vi "ArgoBot_Read.vi"(10 "Open_Cluster":T8) -> (0 "Analog 3":dbl, 1 "Analog 2":dbl, 2 "Analog 1":dbl, 3 "Read_Value":T9 {"Voltage" scale=0.0..6.5; "Analog 1" format="%#_2g"; "Analog 2" format="%#_2g"; "Analog 3" format="%#_2g"; "Loop Rate (Hz)" scale=0.0..50.0}, 4 "GPIO 1 Read":bool, 5 "GPIO 2 Read":bool, 6 "Read_Cluster":T7, 7 "GPIO 3 Read":bool, 8 "Read_Joystick":T10)   [LabVIEW 2016, in "ArgoBotLib.lvlib"]
uses:
  ArgoBotLib.lvlib
  <vilib>/MakerHub/LINX/Private/Type Defs/LINX Ref.ctl
  <vilib>/MakerHub/LINX/Private/Type Defs/Platform.ctl
  <vilib>/MakerHub/LINX/Private/Type Defs/Interface.ctl
  <vilib>/MakerHub/LINX/Private/Device/Type Defs/LINX Device Config.ctl
  <vilib>/MakerHub/LINX/Private/Device/Type Defs/TCP Config.ctl
  <vilib>/MakerHub/LINX/Private/Device/Type Defs/Channels.ctl
  <vilib>/MakerHub/LINX/LMH-LINX.lvlib
  <vilib>/MakerHub/LINX/Private/Device/Device.lvlib
panel:
  # "ArgoBot  Read"
  # "This vi reads the GPIO and Analog channels"
  # "Outputs"
  # "Inputs"
  # "Battery Voltage"
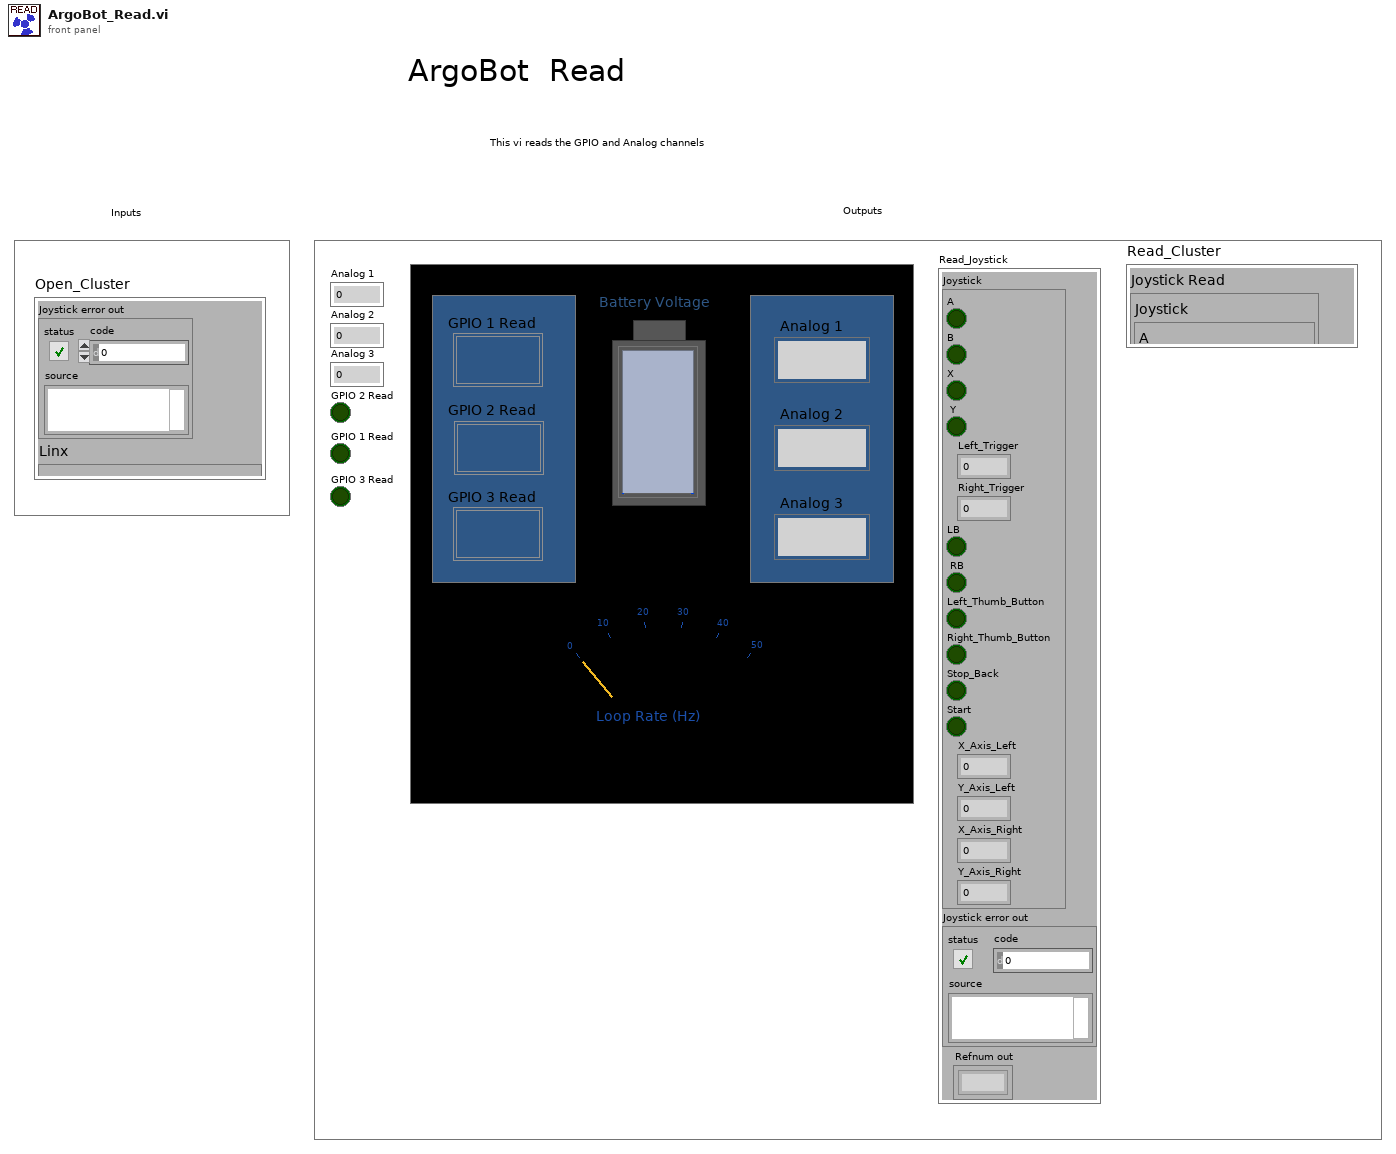
[diagram p1: front panel]
types:
  T1 = typedef "LMH-LINX.lvlib/LINX Ref.ctl" = cluster{"IO":T2, "Interface":T3, "LINX Device Config":T4}
  T2 = typedef "LMH-LINX.lvlib/Platform.ctl" = enum16{"Remote", "Local"}
  T3 = typedef "LMH-LINX.lvlib/Interface.ctl" = enum16{"Serial", "TCP"}
  T4 = typedef "LMH-LINX.lvlib/Device.lvlib/LINX Device Config.ctl" = cluster{"Interface":T3, "COM Port":refnum<visa-resource-name>, "TCP Configuration":T5, "Device Family":u8, "Device ID":u8, "Device Name":string, "TCP Ref":refnum<k5>, "Channels":T6}
  T5 = typedef "LMH-LINX.lvlib/Device.lvlib/TCP Config.ctl" = cluster{"IP Address":string, "Port":u16}
  T6 = typedef "LMH-LINX.lvlib/Channels.ctl" = cluster{"DI":u8[], "DO":u8[], "AI":u8[], "AO":u8[], "PWM":u8[], "QE":u8[], "UART":u8[], "I2C 2":u8[], "SPI":u8[], "CAN":u8[], "Servo":u8[], "AI Ref (V)":dbl, "AI Resolution (Bits)":u8, "AO Ref (V)":dbl, "AO Resolution (Bits)":u8}
  T7 = cluster{"Joystick Read":cluster{"Joystick":cluster{"A":bool, "B":bool, "X":bool, " Y":bool, "Left_Trigger":dbl, "Right_Trigger ":dbl, "LB":bool, " RB":bool, "Left_Thumb_Button":bool, "Right_Thumb_Button":bool, "Stop_Back":bool, "Start":bool, "X_Axis_Left":dbl, "Y_Axis_Left":dbl, "X_Axis_Right":dbl, "Y_Axis_Right":dbl}, "Joystick error out":errorcluster, "Refnum out":refnum<k1>}, "Read Config":cluster{"Read_Config":i32[], "Error Out":errorcluster, "LINX Resource 2":T1}, "Read_Value":cluster{"Analog 1":dbl, "Analog 2":dbl, "Analog 3":dbl, "Voltage":dbl, "GPIO 1 Read":bool, "GPIO 2 Read":bool, "GPIO 3 Read":bool, "Loop Rate (Hz)":u32}, "Joystick error out":errorcluster, "Linx":cluster{"LINX Ref":T1, "Error Out":errorcluster}, "Setup":cluster{"Analog 1 Config":u16, "Analog 2 Config":u16, "Analog 3 Config":u16, "GPIO 1 Config":u16, "GPIO 2 Config":u16, "GPIO 3 Config":u16, "Drive Config":u16, "Motor Mode":u16, "Battery_Config":u16, "LED Config":u16}}
  T8 = cluster{"Joystick error out":errorcluster, "Linx":cluster{"LINX Ref":T1, "Error Out":errorcluster}, "Setup":cluster{"Analog 1 Config":u16, "Analog 2 Config":u16, "Analog 3 Config":u16, "GPIO 1 Config":u16, "GPIO 2 Config":u16, "GPIO 3 Config":u16, "Drive Config":u16, "Motor Mode":u16, "Battery_Config":u16, "LED Config":u16}}
  T9 = cluster{"Analog 1":dbl, "Analog 2":dbl, "Analog 3":dbl, "Voltage":dbl, "GPIO 1 Read":bool, "GPIO 2 Read":bool, "GPIO 3 Read":bool, "Loop Rate (Hz)":u32}
  T10 = cluster{"Joystick":cluster{"A":bool, "B":bool, "X":bool, " Y":bool, "Left_Trigger":dbl, "Right_Trigger ":dbl, "LB":bool, " RB":bool, "Left_Thumb_Button":bool, "Right_Thumb_Button":bool, "Stop_Back":bool, "Start":bool, "X_Axis_Left":dbl, "Y_Axis_Left":dbl, "X_Axis_Right":dbl, "Y_Axis_Right":dbl}, "Joystick error out":errorcluster, "Refnum out":refnum<k1>}
  T11 = cluster{"Read_Config":i32[], "Error Out":errorcluster, "LINX Resource 2":T1}
  T12 = cluster{"A":bool, "B":bool, "X":bool, " Y":bool, "Left_Trigger":dbl, "Right_Trigger ":dbl, "LB":bool, " RB":bool, "Left_Thumb_Button":bool, "Right_Thumb_Button":bool, "Stop_Back":bool, "Start":bool, "X_Axis_Left":dbl, "Y_Axis_Left":dbl, "X_Axis_Right":dbl, "Y_Axis_Right":dbl}
  T13 = cluster{"Analog 1 Config":u16, "Analog 2 Config":u16, "Analog 3 Config":u16, "GPIO 1 Config":u16, "GPIO 2 Config":u16, "GPIO 3 Config":u16, "Drive Config":u16, "Motor Mode":u16, "Battery_Config":u16, "LED Config":u16}
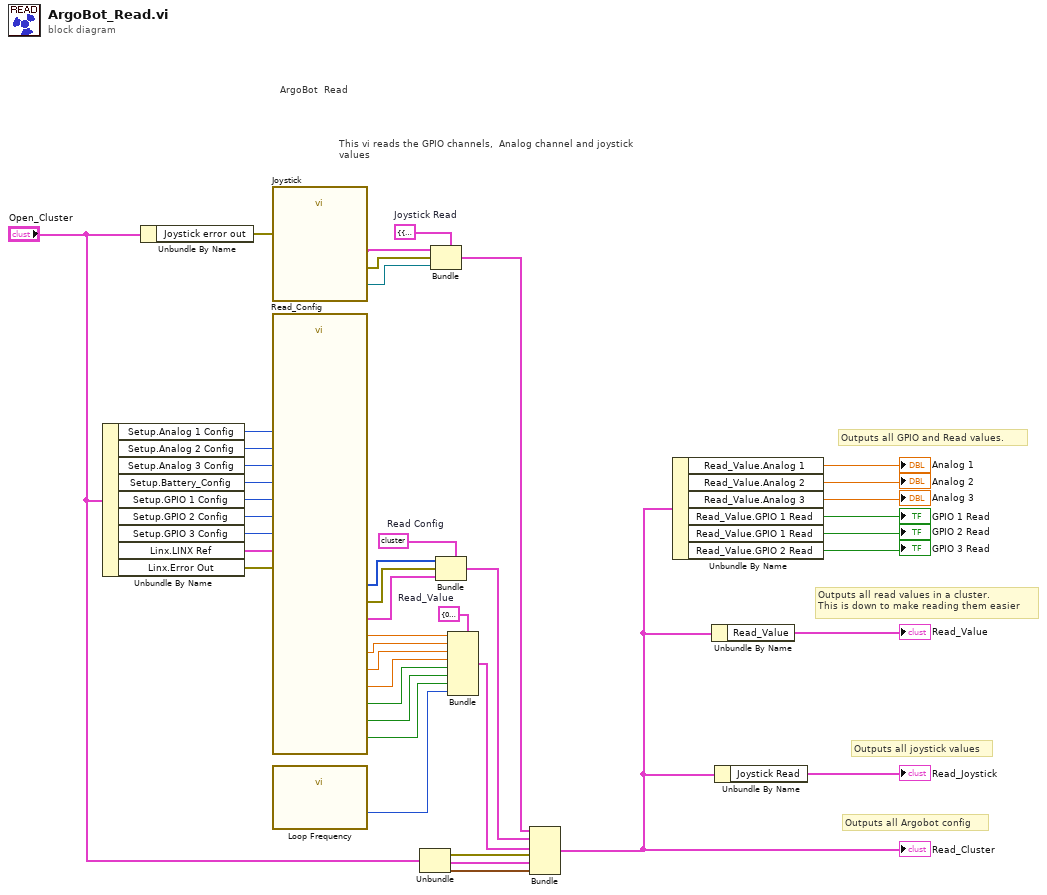
[diagram p0: block diagram]
diagram:
  w12 = T9 {"Analog 1"=0.0, "Analog 2"=0.0, "Analog 3"=0.0, "Voltage"=0.0, "GPIO 1 Read"=FALSE, "GPIO 2 Read"=FALSE, "GPIO 3 Read"=FALSE, "Loop Rate (Hz)"=0}  # Read_Value
  w36 = T11 {"Read_Config"=[], "Error Out"={"status"=FALSE, "code"=0, "source"=""}, "LINX Resource 2"={"IO"=enum."Remote", "Interface"=enum."Serial", "LINX Device Config"={"Interface"=enum."Serial", "COM Port"="", "TCP Configuration"={"IP Address"="", "Port"=0}, "Device Family"=0, "Device ID"=0, "Device Name"="", "TCP Ref"=refnum, "Channels"={"DI"=[], "DO"=[], "AI"=[], "AO"=[], "PWM"=[], "QE"=[], "UART"=[], "I2C 2"=[], "SPI"=[], "CAN"=[], "Servo"=[], "AI Ref (V)"=0.0, "AI Resolution (Bits)"=0, "AO Ref (V)"=0.0, "AO Resolution (Bits)"=0}}}}  # Read Config
  w43 = T10 {"Joystick"={"A"=FALSE, "B"=FALSE, "X"=FALSE, " Y"=FALSE, "Left_Trigger"=0.0, "Right_Trigger "=0.0, "LB"=FALSE, " RB"=FALSE, "Left_Thumb_Button"=FALSE, "Right_Thumb_Button"=FALSE, "Stop_Back"=FALSE, "Start"=FALSE, "X_Axis_Left"=0.0, "Y_Axis_Left"=0.0, "X_Axis_Right"=0.0, "Y_Axis_Right"=0.0}, "Joystick error out"={"status"=FALSE, "code"=0, "source"=""}, "Refnum out"=refnum}  # Joystick Read
  # "Outputs all Argobot config"
  # "Outputs all joystick values"
  # "Outputs all read values in a cluster.  \nThis is down to make reading them easier"
  # "Outputs all GPIO and Read values."
  # "This vi reads the GPIO channels,  Analog channel and joystick values"
  # "ArgoBot  Read"
  n1 = Unbundle By Name("Open_Cluster") -> ("Setup.Analog 1 Config"=w11:u16, "Setup.Analog 2 Config"=w10:u16, "Setup.Analog 3 Config"=w9:u16, "Setup.Battery_Config"=w8:u16, "Setup.GPIO 1 Config"=w7:u16, "Setup.GPIO 2 Config"=w6:u16, "Setup.GPIO 3 Config"=w5:u16, "Linx.LINX Ref"=w21:T1, "Linx.Error Out"=w20:errorcluster)
  n2 = Unbundle By Name("Open_Cluster") -> ("Joystick error out"=w1:errorcluster)
  n3 = call "Joystick.vi"("Joystick error in"=w1) -> ("Joystick error out"=w41:errorcluster, "Joystick"=w40:T12, "Refnum out"=w42:refnum<k1>)  [unwired: 8 in]
  n4 = call "Read_Config.vi"("GPIO 1 Config"=w7, "GPIO 2 Config"=w6, "GPIO 3 Config"=w5, "Battery_Config"=w8, "Analog 1 Config"=w11, "Analog 2 Config"=w10, "Analog 3 Config"=w9, "Error In"=w20, "LINX Resource"=w21) -> ("Read_Config"=w24:i32[], "Voltage"=w3:dbl, "GPIO 1 Read"=w17:bool, "Analog 2"=w38:dbl, "GPIO 2 Read"=w18:bool, "Analog 3"=w39:dbl, "GPIO 3 Read"=w19:bool, "Error Out"=w23:errorcluster, "Analog 1"=w37:dbl, "LINX Resource 2"=w22:T1)  [unwired: 9 in]
  n5 = call <vilib>:"Loop Frequency.vi"() -> ("Loop Rate (Hz)"=w16:u32)
  n6 = Unbundle("Open_Cluster") -> ("Joystick error out"=w35:errorcluster, "Linx"=w34:cluster{"LINX Ref":T1, "Error Out":errorcluster}, "Setup"=w33:T13)
  n7 = Bundle ("Joystick Read")(cluster=w43, "Joystick"=w40, "Joystick error out"=w41, "Refnum out"=w42) -> (w13:T10)
  n8 = Bundle ("Read Config")(cluster=w36, "Read_Config"=w24, "Error Out"=w23, "LINX Resource 2"=w22) -> (w14:T11)
  n9 = Bundle ("Read Config")(cluster=w12, "Analog 1"=w37, "Analog 2"=w38, "Analog 3"=w39, "Voltage"=w3, "GPIO 1 Read"=w17, "GPIO 2 Read"=w18, "GPIO 3 Read"=w19, "Loop Rate (Hz)"=w16) -> (w15:T9)
  n10 = Bundle("Joystick Read"=w13, "Read Config"=w14, "Read_Value"=w15, "Joystick error out"=w35, "Linx"=w34, "Setup"=w33) -> (w25:T7)  [unwired: 1 in]
  "Read_Cluster" <- w25
  n11 = Unbundle By Name(w25) -> ("Read_Value.Analog 1"=→"Analog 1":dbl, "Read_Value.Analog 2"=→"Analog 2":dbl, "Read_Value.Analog 3"=→"Analog 3":dbl, "Read_Value.GPIO 1 Read"=→"GPIO 1 Read":bool, "Read_Value.GPIO 1 Read"=→"GPIO 2 Read":bool, "Read_Value.GPIO 2 Read"=→"GPIO 3 Read":bool)
  n12 = Unbundle By Name(w25) -> ("Read_Value"=→"Read_Value":T9)
  n13 = Unbundle By Name(w25) -> ("Joystick Read"=→"Read_Joystick":T10)
